vi "Init.vi"(10 "Input":T1) -> (3 "TEMPLATE Msg Input out":refnum<class "TEMPLATE Msg Input.lvclass">)   [LabVIEW 2020, in "_Template.lvlib" / "Templates.lvlib" / "TEMPLATE jettl Msg.lvlib" / "TEMPLATE Msg Input.lvlib" / "TEMPLATE Msg Input.lvclass"]
uses:
  TEMPLATE Msg Input.lvclass
  TEMPLATE Msg Input.lvclass/TEMPLATE Msg Input.ctl
  Input.ctl
  TEMPLATE jettl Msg.lvlib
panel:
  # "This front panel should not be manipulated."
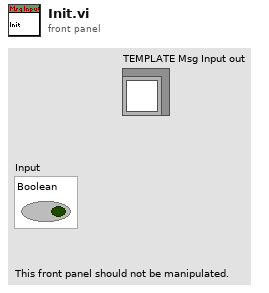
[diagram p1: front panel]
types:
  T1 = typedef "_Template.lvlib/Templates.lvlib/TEMPLATE jettl Msg.lvlib/Input.ctl" = cluster{"Boolean":bool}
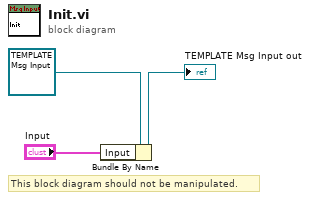
[diagram p0: block diagram]
diagram:
  # "This block diagram should not be manipulated."
  n1 = Bundle By Name(cluster=refnum<class "TEMPLATE Msg Input.lvclass"> refnum ("Object"), "Input"="Input") -> (→"TEMPLATE Msg Input out":refnum<class "TEMPLATE Msg Input.lvclass">)
